vi "destroy.vi"(8 "error in (no error)":errorcluster, 11 "base view in":refnum<class "base view.lvclass">) -> (0 "error out":errorcluster, 3 "base view out":refnum<class "base view.lvclass">)   [LabVIEW 2022 SP3, in "base view.lvclass"]
uses:
  base view.lvclass
  base view.lvclass/base view.ctl
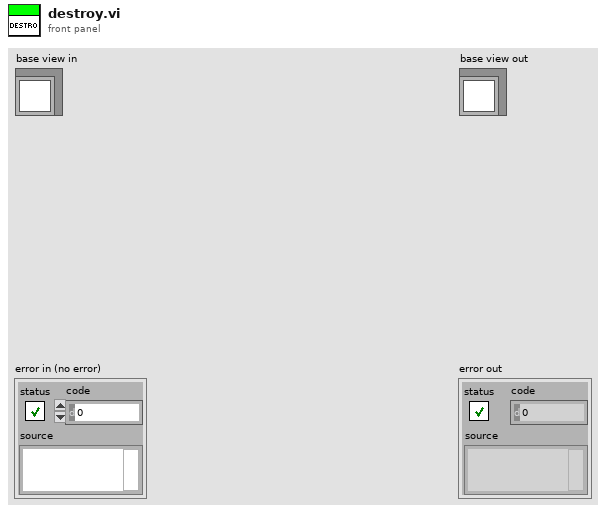
[diagram p1: front panel]
types:
  T1 = typedef "base view.lvclass/Data.ctl" = cluster{"View Refnum":refnum<vi>, "Wrapped View Refnum":refnum<vi>, "Events":T2}
  T2 = typedef "base view.lvclass/Events.ctl" = cluster{"Open":refnum<user-event>, "Close":refnum<user-event>, "Hide":refnum<user-event>}
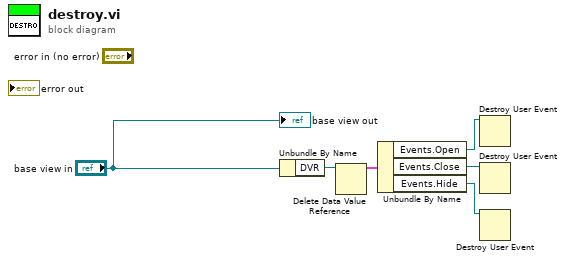
[diagram p0: block diagram]
diagram:
  n1 = Unbundle By Name("base view in") -> ("DVR"=w5:refnum<data-value>)
  n2 = Delete Data Value Reference(data value reference=w5) -> (data value=w4:T1)  [unwired: 1 in, 1 out]
  n3 = Unbundle By Name(w4) -> ("Events.Open"=w3:refnum<user-event>, "Events.Close"=w2:refnum<user-event>, "Events.Hide"=w1:refnum<user-event>)
  n4 = Destroy User Event(user event=w3) -> ()  [unwired: 1 in, 1 out]
  n5 = Destroy User Event(user event=w2) -> ()  [unwired: 1 in, 1 out]
  n6 = Destroy User Event(user event=w1) -> ()  [unwired: 1 in, 1 out]
  "base view out" <- "base view in"
